vi "uNotify Update.vi"(8 "error in (no error)":errorcluster, 9 "Destination uMsg":refnum<class "uMsg.lvclass">, 10 "uTransport":refnum<class "uTransport.lvclass">, 11 "uNotifyMode in":refnum<class "uNotifyMode.lvclass">) -> (0 "error out":errorcluster)   [LabVIEW 2021, in "uFramework.lvlib" / "uNotifyMode.lvclass"]
uses:
  uNotifyMode.lvclass
  uNotifyMode.lvclass/uNotifyMode.ctl
  uTransport/uTransport.lvclass
  uTransport_uActor/uTransport_uActor.lvclass
  uTransport_Event/uTransport_Event.lvclass
  uTransport_Queue/uTransport_Queue.lvclass
  uMsg/uMsg.lvclass
  uActor/uActor.lvclass
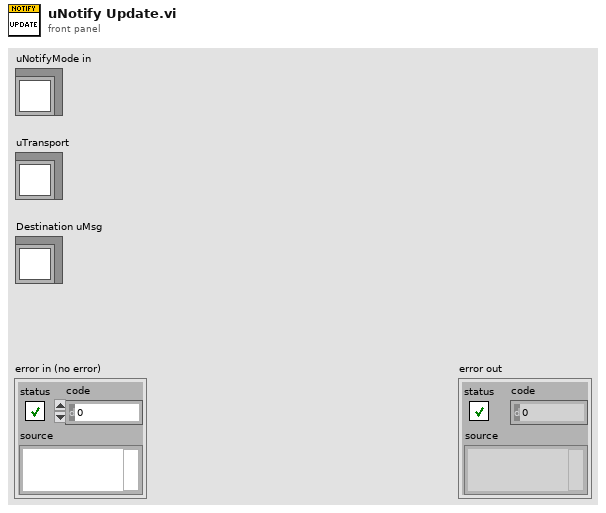
[diagram p1: front panel]
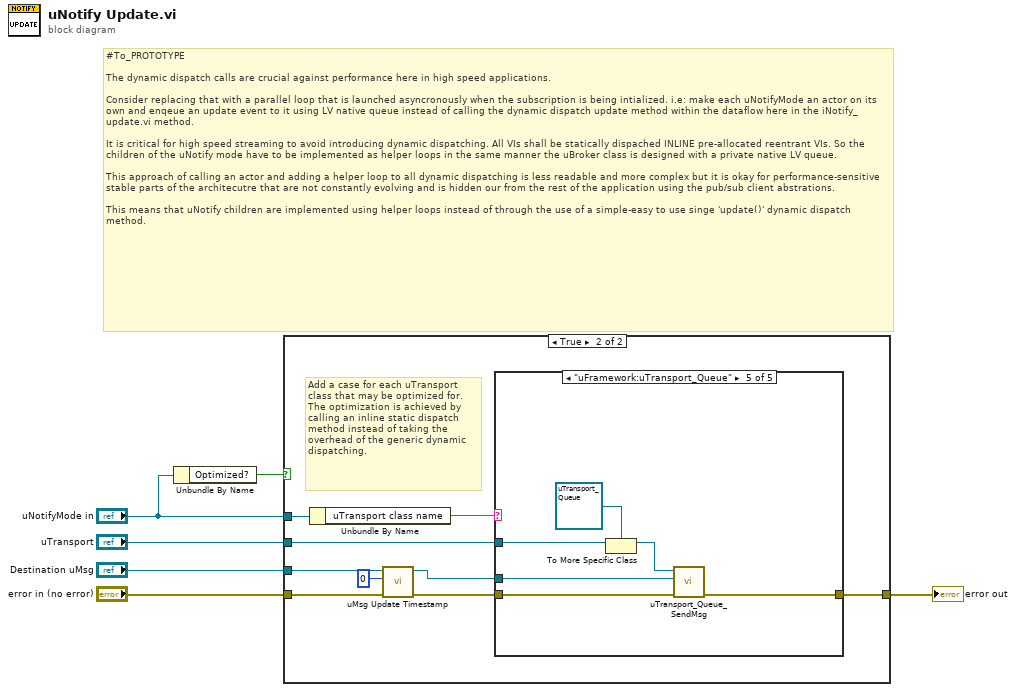
[diagram p0: block diagram]
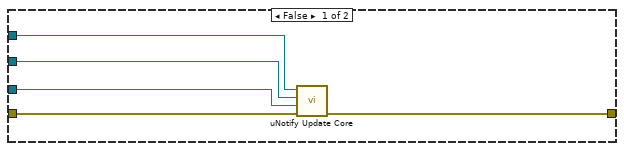
[diagram p2: hidden frame]
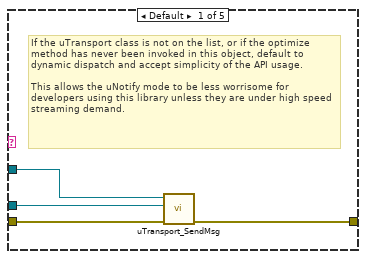
[diagram p3: hidden frame]
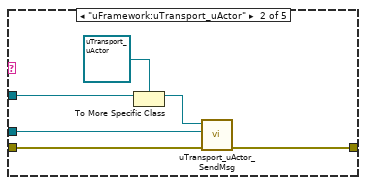
[diagram p4: hidden frame]
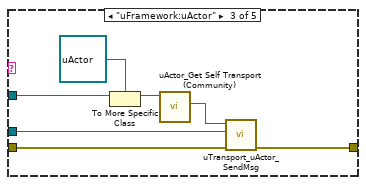
[diagram p5: hidden frame]
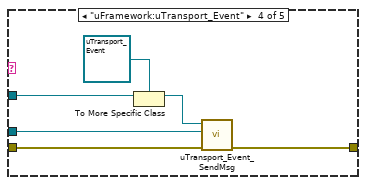
[diagram p6: hidden frame]
diagram:
  # "#To_PROTOTYPE\n\nThe dynamic dispatch calls are crucial against performance here in high speed applications.\n\nConsider replacing that with a parallel loop that is launched asyncronously when the subscription is being intialized. i.e: make each uNotifyMode an actor on its own and enqeue an update event to it using LV native queue instead of calling the dynamic dispatch update method within the dataflow here in the iNotify_update.vi method.\n\nIt is critical for high speed streaming to avoid introducing dynamic dispatching. All VIs shall be statically dispached INLINE pre-allocated reentrant VIs. So the children of the uNotify mode have to be implemented as helper loops in the same manner the uBroker class is designed with a private native LV queue.\n\nThis approach of calling an actor and adding a helper loop to all dynamic dispatching is less readable and more complex but it is okay for performance-sensitive stable parts of the architecutre that are not constantly evolving and is hidden our from the rest of the application using the pub/sub client abstrations.\n\nThis means that uNotify children are implemented using helper loops instead of through the use of a simple-easy to use singe 'update()' dynamic dispatch method."
  n1 = Unbundle By Name("uNotifyMode in") -> ("Optimized?"=w1:bool)
  n2 = case shown="True" w1 {
    tunnel: "error in (no error)" -> [w11 w16]
    tunnel: [w10 w15] -> w5
    tunnel: "Destination uMsg" -> [w8 w14]
    tunnel: "uTransport" -> [w7 w13]
    tunnel: "uNotifyMode in" -> [w9 w12]
    frame False {
      n3 = call-dynamic "uNotify Update Core.vi"("error in (no error)"=w11, "Destination uMsg"=w8, "uTransport"=w7, "uNotifyMode in"=w9) -> ("error out"=w10:errorcluster)  [unwired: 7 in]
    }
    frame True {
      # "Add a case for each uTransport class that may be optimized for. The optimization is achieved by calling an inline static dispatch method instead of taking the overhead of the generic dynamic dispatching."
      n4 = Unbundle By Name(w12) -> ("uTransport class name"=w19:string)
      n5 = call "uMsg Update Timestamp.vi"("error in (no error)"=w16, "Timestamp"=u32 0, "uMsg in"=w14) -> ("error out"=w18:errorcluster, "uMsg out"=w17:refnum<class "uMsg.lvclass">)  [unwired: 7 in]
      n6 = case shown="\"uFramework:uTransport_Queue\"" w19 {
        tunnel: w18 -> [w24 w30 w37 w41 w47]
        tunnel: [w23 w28 w35 w40 w46] -> w15
        tunnel: w17 -> [w22 w25 w33 w38 w44]
        tunnel: w13 -> [w21 w29 w36 w39 w45]
        frame Default {
          # "If the uTransport class is not on the list, or if the optimize method has never been invoked in this object, default to dynamic dispatch and accept simplicity of the API usage.\n\nThis allows the uNotify mode to be less worrisome for developers using this library unless they are under high speed streaming demand."
          n7 = call "uTransport_SendMsg.vi"("error in (no error)"=w24, "Msg"=w22, "uTransport in"=w21) -> ("error out"=w23:errorcluster)  [unwired: 7 in, 1 out]
        }
        frame "uFramework:uTransport_uActor" {
          n8 = To More Specific Class(target class=refnum<class "uTransport_uActor.lvclass"> refnum, reference=w29) -> (specific class reference=w26:refnum<class "uTransport_uActor.lvclass">)  [unwired: 1 in, 1 out]
          n9 = call "uTransport_uActor_SendMsg.vi"("error in (no error)"=w30, "Msg"=w25, "uTransport_uActor in"=w26) -> ("error out"=w28:errorcluster)  [unwired: 8 in]
        }
        frame "uFramework:uActor" {
          n10 = To More Specific Class(target class=refnum<class "uActor.lvclass"> refnum, reference=w36) -> (specific class reference=w32:refnum<class "uActor.lvclass">)  [unwired: 1 in, 1 out]
          n11 = call "uActor_Get Self Transport (Community).vi"("uActor in"=w32) -> ("Actor Transport"=w31:refnum<class "uTransport_uActor.lvclass">)  [unwired: 9 in, 1 out]
          n12 = call "uTransport_uActor_SendMsg.vi"("error in (no error)"=w37, "Msg"=w33, "uTransport_uActor in"=w31) -> ("error out"=w35:errorcluster)  [unwired: 8 in]
        }
        frame "uFramework:uTransport_Event" {
          n13 = To More Specific Class(target class=refnum<class "uTransport_Event.lvclass"> refnum, reference=w39) -> (specific class reference=w42:refnum<class "uTransport_Event.lvclass">)  [unwired: 1 in, 1 out]
          n14 = call "uTransport_Event_SendMsg.vi"("error in (no error)"=w41, "Msg"=w38, "uTransport_Event in"=w42) -> ("error out"=w40:errorcluster)  [unwired: 7 in, 1 out]
        }
        frame "uFramework:uTransport_Queue" {
          n15 = To More Specific Class(target class=refnum<class "uTransport_Queue.lvclass"> refnum, reference=w45) -> (specific class reference=w48:refnum<class "uTransport_Queue.lvclass">)  [unwired: 1 in, 1 out]
          n16 = call "uTransport_Queue_SendMsg.vi"("error in (no error)"=w47, "Msg"=w44, "uTransport_Queue in"=w48) -> ("error out"=w46:errorcluster)  [unwired: 7 in, 1 out]
        }
      }
    }
  }
  "error out" <- w5
